vi "testdistToObs.vi"() -> ()   [LabVIEW 2013]
uses:
  Data/TypeDefs/UTM Location.ctl
panel:
  out "Distance between boat and segment":dbl
  in  "Boat Point":T1 {"North" format="%#_10f"; "East" format="%#_8f"}
  in  "Segment Point 2":T1 {"North" format="%#_10f"; "East" format="%#_8f"}
  in  "Segment Point 1":T1 {"North" format="%#_10f"; "East" format="%#_8f"}
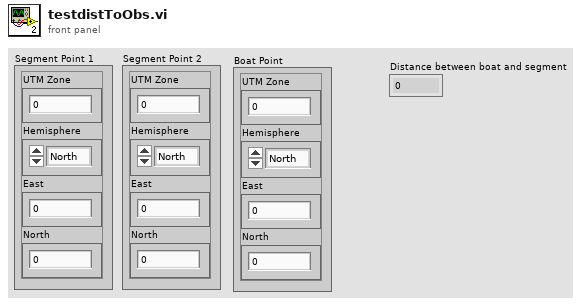
[diagram p1: front panel]
types:
  T1 = typedef "UTM Location.ctl" = cluster{"UTM Zone":dbl, "Hemisphere":enum16{"North", "South"}, "East":dbl, "North":dbl}
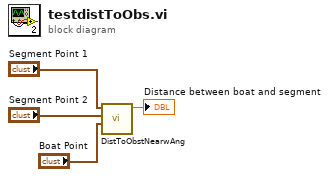
[diagram p0: block diagram]
diagram:
  n1 = call "DistToObstNearwAng.vi"("Boat Point"="Boat Point", "Segment Point 2"="Segment Point 2", "Segment Point 1"="Segment Point 1") -> ("Distance between boat and segment"=→"Distance between boat and segment":dbl)  [unwired: 7 in, 1 out]
